vi "Handle Error.vi"(8 "error in":errorcluster) -> (0 "error out":errorcluster)   [LabVIEW 2020, in "Error Handler.lvlib"]
doc: "Holds reference to communication structure need by the current module both for internal and external use"
uses:
  Error Handler.lvlib
  Controller/Controls/Application Modules.ctl
  Controller/Controller.lvlib
  Controls/Error Message Object.ctl
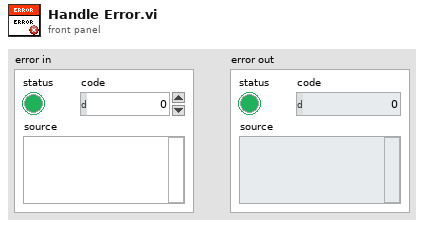
[diagram p1: front panel]
types:
  T1 = typedef "Controller.lvlib/Application Modules.ctl" = enum16{"Controller", "Error Module", "User Console", "Display Console", "Sensor Interface"}
  T2 = typedef "Error Handler.lvlib/Error Message Object.ctl" = cluster{"Source Module":T1, "Error":errorcluster}
  T3 = enum16{"Load References", "Release References", "Get References"}
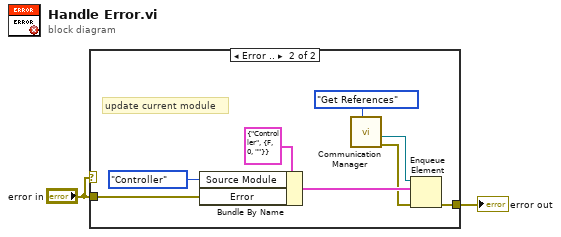
[diagram p0: block diagram]
diagram:
  n1 = case shown="Error .." "error in" {
    tunnel: [w3 w7] -> w2
    tunnel: "error in" -> [w3 w6]
    frame No Error {
    }
    frame Error {
      # "update current module"
      n2 = Bundle By Name(cluster=T2 {"Source Module"=enum."Controller", "Error"={"status"=FALSE, "code"=0, "source"=""}} ("element"), "Source Module"=Application_Modules."Controller", "Error"=w6) -> (w8:T2)
      n3 = call "Communication Manager.vi"("Mode"=T3."Get References") -> ("error out"=w4:errorcluster, "Error Queue Out"=w10:refnum<queue>)  [unwired: 8 in, 1 out]
      n4 = Enqueue Element(queue=w10, element=w8, error in (no error)=w4) -> (error out=w7:errorcluster)  [unwired: 1 in, 2 out]
    }
  }
  "error out" <- w2
